vi "PixyAllDetect.vi"(8 "error in (no error)":errorcluster, 11 "String":string) -> (0 "error out":errorcluster, 3 "output array":bool[](array[boolean]))   [LabVIEW 2017]
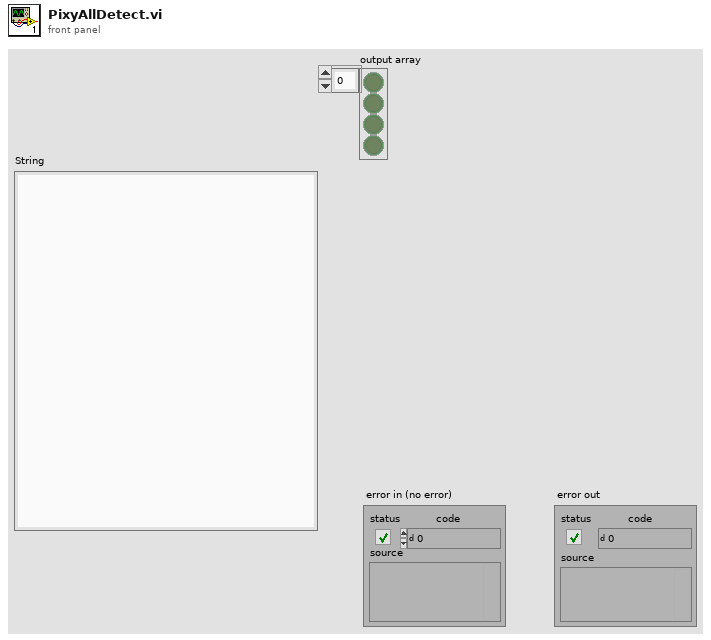
[diagram p1: front panel]
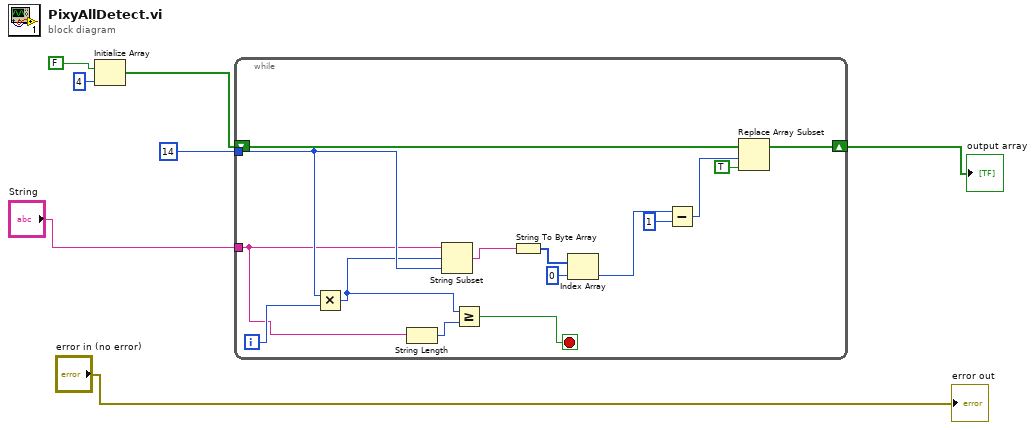
[diagram p0: block diagram]
diagram:
  n1 = Initialize Array(FALSE, 4 ("dimension size")) -> (w4:bool[])
  n2 = while {
    tunnel: 14 ("length (rest)") -> [w21]
    shift-right: [w9] -> w3
    shift-left: w4 -> [w14]
    tunnel: "String" -> [w8]
    i -> [w22]
    stop <- w18 stop-if-true
    n3 = Multiply(x=w21, y=w22) -> (x*y=w20:i32)
    n4 = String Length(string=w8) -> (length=w19:i32)
    n5 = String Subset(string=w8, offset (0)=w20, length (rest)=w21) -> (substring=w17:string)
    n6 = Greater Or Equal?(x=w20, y=w19) -> (x >= y?=w18:bool)
    n7 = String To Byte Array(string=w17) -> (unsigned byte array=w16:u8[])
    n8 = Index Array(array=w16, index=0) -> (element=w13:u8)
    n9 = Subtract(x=w13, y=u8 1) -> (x-y=w11:u8)
    n10 = Replace Array Subset(array=w14, new element=TRUE ("new element/subarray"), index=w11) -> (w9:bool[])
  }
  "output array" <- w3
  "error out" <- "error in (no error)"
